vi "errorToCluster.vi"(0 "error code":T2, 2 "error message (\"\")":string, 5 "error in (no error)":errorcluster, 8 "show call chain? (True)":bool=TRUE, 9 "severity (Error)":T1=enum."Error") -> (19 "error out":errorcluster)   [LabVIEW 2014, in "HGF_Auxiliary.lvlib"]
doc: "Converts error code and severity information to an error cluster. This VI is useful when you return HGF_Error codes."
uses:
  HGF_Auxiliary.lvlib
  ErrorCode.ctl
  Severity.ctl
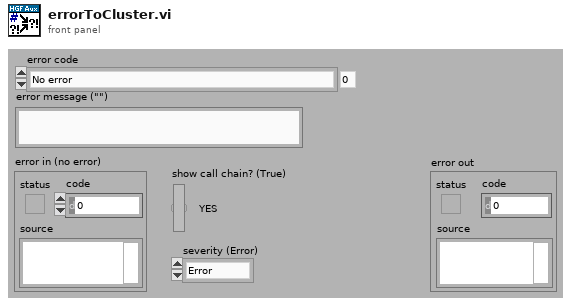
[diagram p1: front panel]
types:
  T1 = typedef "HGF_Auxiliary.lvlib/Severity.ctl" = enum16{"Info", "Warning", "Fault", "Error", "Fatal"}
  T2 = typedef "HGF_Auxiliary.lvlib/ErrorCode.ctl" = enum32{"No error", "Function not supported.", "This VI is for friends only.", "Reference object aready exisits.", "Parameter out of range.", "Not a rendezvous.", "Invalid notifier reference.", "Invalid queue reference.", "Self-Test not supported.", "Reset not supported.", "IDN query not supported.", "Error query not supported.", "Incorrect addressee.", "Object already exists.", "No class name specified", "Driver not supported", "Attribute is not writable"}
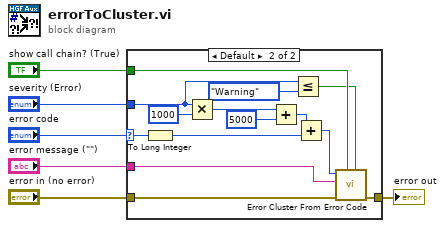
[diagram p0: block diagram]
diagram:
  n1 = case shown="Default" "error code" {
    selector: "error code" -> [_ w12]
    tunnel: "error message (\"\")" -> [_ w8]
    tunnel: "error in (no error)" -> [w7 w10]
    tunnel: "show call chain? (True)" -> [_ w20]
    tunnel: [w7 w19] -> w3
    tunnel: "severity (Error)" -> [_ w9]
    frame "No error" {
    }
    frame Default {
      n2 = To Long Integer(number=w12) -> (32bit integer=w11:i32)
      n3 = Multiply(x=w9, y=1000) -> (x*y=w13:i32)
      n4 = Add(x=w13, y=5000) -> (x+y=w17:i32)
      n5 = Less Or Equal?(x=w9, y=Severity."Warning" ("HGF_Severity")) -> (x <= y?=w15:bool)
      n6 = Add(x=w17, y=w11) -> (x+y=w21:i32)
      n7 = call <vilib>:"Error Cluster From Error Code.vi"("is warning? (False)"=w15, "show call chain? (False)"=w20, "error in (no error)"=w10, "error message (\"\")"=w8, "error code (0)"=w21) -> ("error out"=w19:errorcluster)  [unwired: 4 out]
    }
  }
  "error out" <- w3
